vi "int2sortablestring.vi"(10 "int":u32) -> (2 "tens-sortable-string":string)   [LabVIEW 2017]
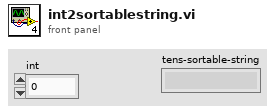
[diagram p1: front panel]
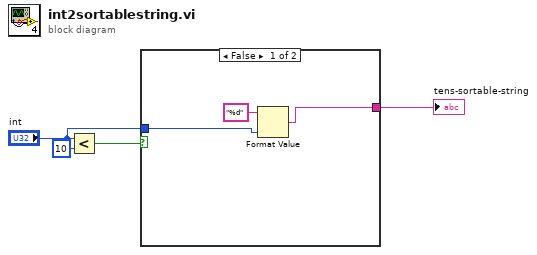
[diagram p0: block diagram]
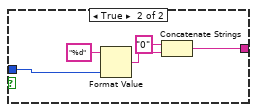
[diagram p2: hidden frame]
diagram:
  n1 = Less?(x="int", y=u32 10) -> (x < y?=w3:bool)
  n2 = case shown="False" w3 {
    tunnel: "int" -> [w6 w11]
    tunnel: [w5 w8] -> w1
    frame False {
      n3 = Format Value(format string="%d", value (0)=w6) -> (output string=w5:string)  [unwired: 1 in]
    }
    frame True {
      n4 = Format Value(format string="%d", value (0)=w11) -> (output string=w10:string)  [unwired: 1 in]
      n5 = Concatenate Strings("0" ("string"), w10) -> (w8:string)
    }
  }
  "tens-sortable-string" <- w1
